vi "Parse Results (single).vi"(6 "Type":T1, 8 "error in (no error)":errorcluster, 9 "Reference Channel":i32=1, 10 "AI Channel":i32=1, 11 "Results (Dictionary)":cluster{"key":string, "value":dbl}[](array[cluster])) -> (0 "error out":errorcluster, 1 "Name":string, 2 "Data":dbl, 3 "Results (Dictionary)":cluster{"key":string, "value":dbl}[](array[cluster]))   [LabVIEW 2019, in "Instrument.LockinAPI.lvclass"]
uses:
  Instrument.LockinAPI.lvclass
  Typedefs/Results Type--Enum.ctl
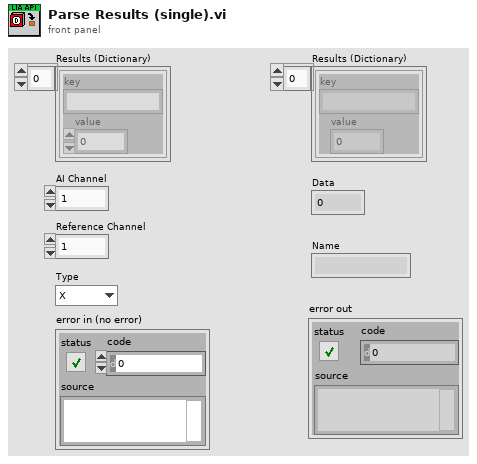
[diagram p1: front panel]
types:
  T1 = typedef "Instrument.LockinAPI.lvclass/Results Type--Enum.ctl" = enum16{"X", "Y", "R", "Theta", "Mean"}
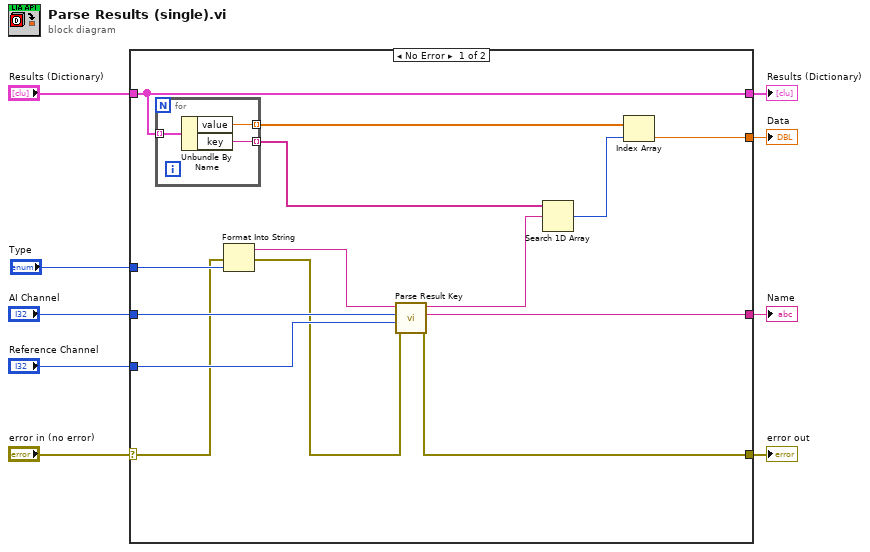
[diagram p0: block diagram]
diagram:
  n1 = case shown="No Error" "error in (no error)" {
    selector: "error in (no error)" -> [w11 w27]
    tunnel: [w19 _] -> w9
    tunnel: "Type" -> [w13 _]
    tunnel: "Results (Dictionary)" -> [w22 w28]
    tunnel: [w15 _] -> w1
    tunnel: [w14 w27] -> w5
    tunnel: [w22 w28] -> w4
    tunnel: "Reference Channel" -> [w17 _]
    tunnel: "AI Channel" -> [w18 _]
    frame No Error {
      n2 = for {
        tunnel: [w26] -> w21 mode=indexing
        tunnel: [w25] -> w23 mode=indexing
        tunnel: w22 -> [w24] mode=indexing
        n3 = Unbundle By Name(w24) -> ("value"=w26:dbl, "key"=w25:string)
      }
      n4 = Format Into String(error in=w11, w13) -> (resulting string=w12:string, error out=w10:errorcluster)  [unwired: 2 in]
      n5 = call "Parse Result Key.vi"("error in (no error)"=w10, "Ref Channel"=w17, "AI Channel"=w18, "Datatype"=w12) -> ("error out"=w14:errorcluster, "Label"=w15:string, "Key"=w16:string)  [unwired: 5 in]
      n6 = Search 1D Array(1D array=w23, element=w16) -> (index of element=w20:i32)  [unwired: 1 in]
      n7 = Index Array(array=w21, index=w20) -> (element=w19:dbl)
    }
    frame Error {
    }
  }
  "Data" <- w9
  "Results (Dictionary)" <- w4
  "Name" <- w1
  "error out" <- w5
